vi "Stop Core.vi"(10 "final error code":i32, 11 "ActorCountsMessageCycles in":refnum<class "ActorCountsMessageCycles.lvclass">) -> (3 "ActorCountsMessageCycles out":refnum<class "ActorCountsMessageCycles.lvclass">)   [LabVIEW 2017, in "ActorCountsMessageCycles.lvclass"]
doc: "(<B>Filename</B>: Actor Framework.lvlib:Actor.lvclass:Stop Core.vi)\n\nDefines what the actor does before it stops. Use the <B>final error code</B> input to determine whether the actor shut down in response to an error.\n\nBy default, this method does nothing. A descendant class may override it to define behavior, such as shutting down any processes the actor initiated in its override of the Actor Core method."
uses:
  ActorCountsMessageCycles.lvclass
  ActorCountsMessageCycles.lvclass/ActorCountsMessageCycles.ctl
  <vilib>/ActorFramework/Actor/Actor.lvclass
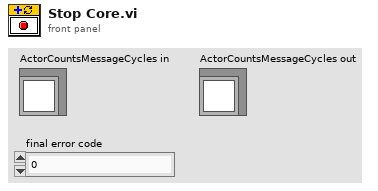
[diagram p1: front panel]
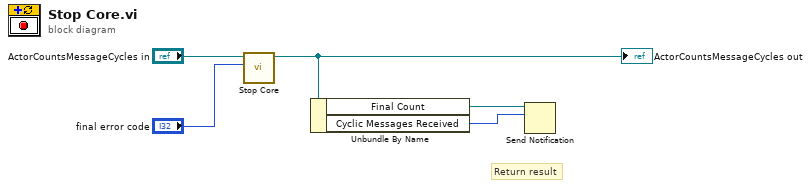
[diagram p0: block diagram]
diagram:
  # "Return result"
  n1 = call-parent "Stop Core.vi"("final error code"="final error code", "Actor in"="ActorCountsMessageCycles in") -> ("Actor out"=w3:refnum<class "ActorCountsMessageCycles.lvclass">)  [unwired: 9 in]
  "ActorCountsMessageCycles out" <- w3
  n2 = Unbundle By Name(w3) -> ("Final Count"=w2:refnum<notifier>, "Cyclic Messages Received"=w1:u32)
  n3 = Send Notification(notification=w1, notifier=w2) -> ()  [unwired: 1 in, 2 out]
